vi "Load_waveform_file.vi"(10 "N":i32, 11 "Enable limit = True":bool=TRUE) -> (1 "Loop ?":i32, 2 "selected path":path, 3 "first waveform in record":waveform(dbl), 5 "Sample_Rate":dbl)   [LabVIEW 2017]
uses:
  <vilib>/Waveform/WDTFileIO.llb/Read Waveform from File.vi
  <vilib>/Waveform/WDTOps.llb/WDT Append Waveforms DBL.vi
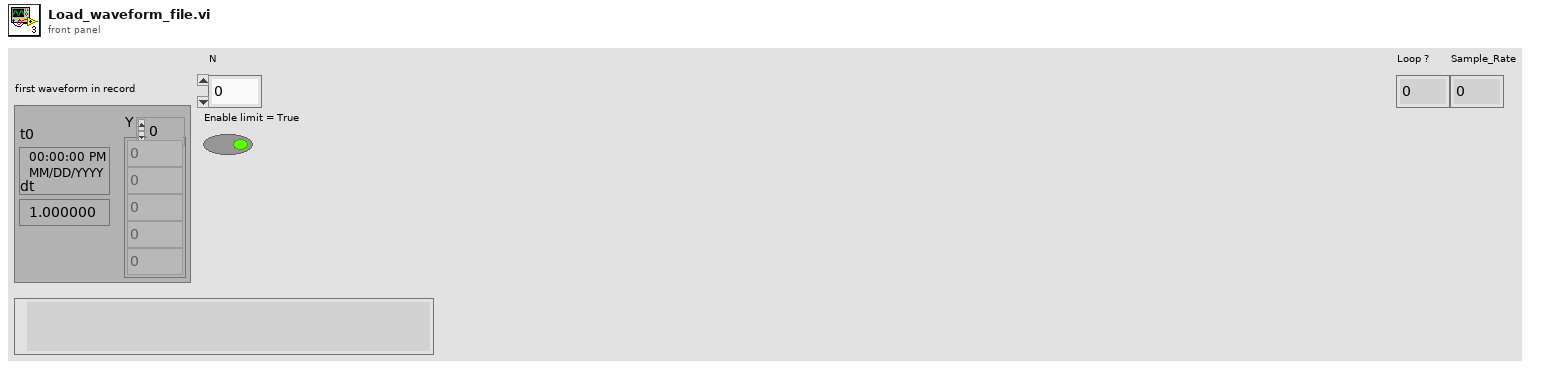
[diagram p1: front panel]
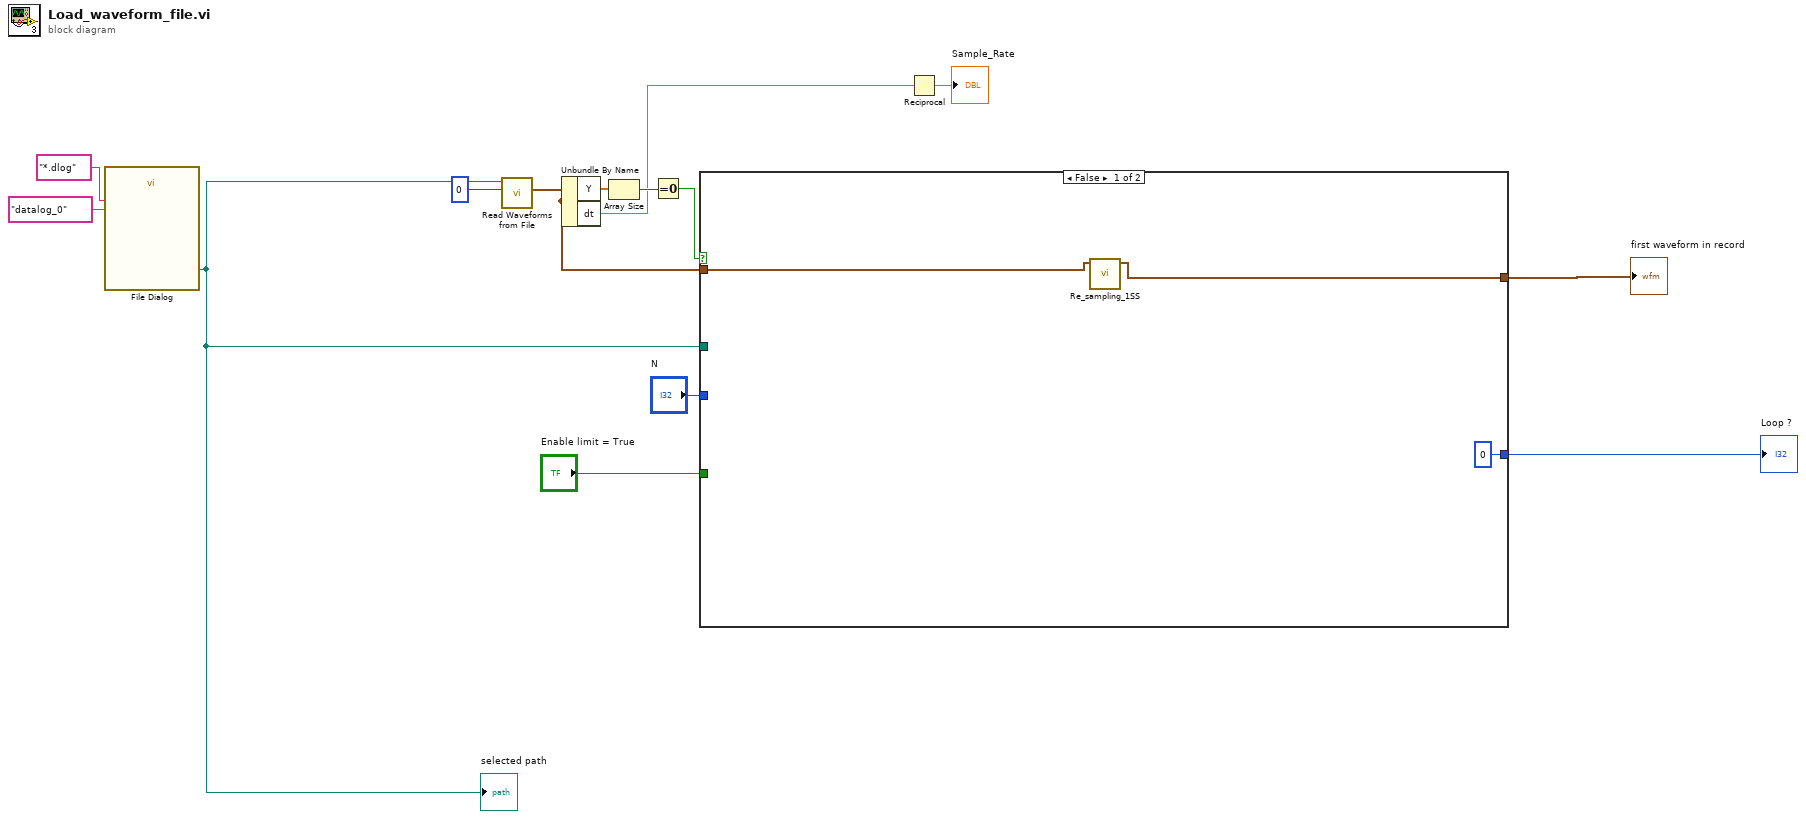
[diagram p0: block diagram]
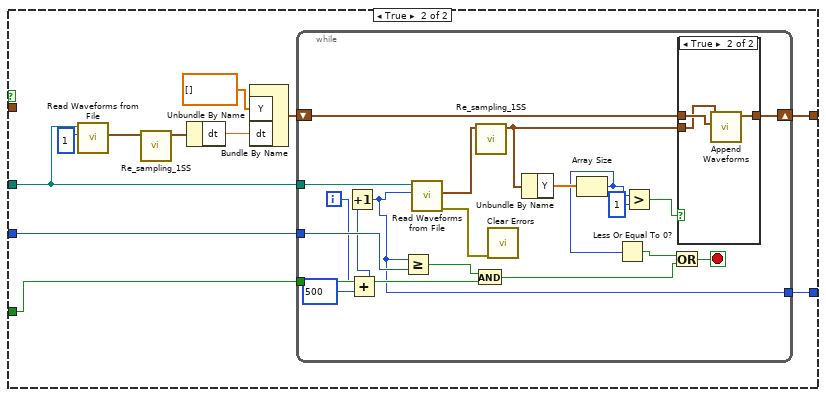
[diagram p2: hidden frame]
diagram:
  n1 = call "File Dialog"("pattern (all files)"="*.dlog", "pattern label"="datalog_0") -> ("selected path"=w11:path)  [unwired: 10 in, 3 out]
  "selected path" <- w11
  n2 = call-poly <vilib>:"Read Waveforms from File.vi"("offset (records:0)"=0, "file path (dialog if empty)"=w11) -> ("first waveform in record"=w3:waveform(dbl))  [unwired: 4 in, 3 out]
  n3 = Unbundle By Name(w3) -> ("Y"=w12:dbl[], "dt"=w2:dbl)
  n4 = Array Size(array=w12) -> (size(s)=w13:i32)
  n5 = Equal To 0?(x=w13) -> (x = 0?=w14:bool)
  n6 = case shown="False" w14 {
    tunnel: [w15 w28] -> w9
    tunnel: w11 -> [_ w23]
    tunnel: "N" -> [_ w22]
    tunnel: "Enable limit = True" -> [_ w21]
    tunnel: [0 w18] -> w4
    tunnel: w3 -> [w16 _]
    frame False {
      n7 = call "Re_sampling_1SS.vi"("Waveform_main"=w16) -> ("Waveform"=w15:waveform(dbl))  [unwired: 10 in]
    }
    frame True {
      n8 = call-poly <vilib>:"Read Waveforms from File.vi"("offset (records:0)"=1, "file path (dialog if empty)"=w23) -> ("first waveform in record"=w20:waveform(dbl))  [unwired: 4 in, 3 out]
      n9 = call "Re_sampling_1SS.vi"("Waveform_main"=w20) -> ("Waveform"=w19:waveform(dbl))  [unwired: 10 in]
      n10 = Unbundle By Name(w19) -> ("dt"=w25:dbl)
      n11 = Bundle By Name("Y"=dbl[] [], "dt"=w25) -> (w24:waveform(dbl))  [unwired: 1 in]
      n12 = while {
        shift-right: [w48] -> w28
        shift-left: w24 -> [w44]
        tunnel: w23 -> [w47]
        tunnel: w22 -> [w43]
        tunnel: w21 -> [w40]
        tunnel: [w33] -> w18
        i -> [w31]
        stop <- w42 stop-if-true
        n13 = Add(x=w31, y=500) -> (x+y=w29:i32)
        n14 = Increment(x=w29) -> (x+1=w33:i32)
        n15 = Greater Or Equal?(x=w33, y=w43) -> (x >= y?=w41:bool)
        n16 = call-poly <vilib>:"Read Waveforms from File.vi"("offset (records:0)"=w33, "file path (dialog if empty)"=w47) -> ("error out"=w45:errorcluster, "first waveform in record"=w32:waveform(dbl))  [unwired: 4 in, 2 out]
        n17 = And(x=w41, y=w40) -> (x .and. y?=w39:bool)
        n18 = call "Re_sampling_1SS.vi"("Waveform_main"=w32) -> ("Waveform"=w38:waveform(dbl))  [unwired: 10 in]
        n19 = call <vilib>:"Clear Errors.vi"("error in (no error)"=w45) -> ()  [unwired: 5 in, 2 out]
        n20 = Unbundle By Name(w38) -> ("Y"=w46:dbl[])
        n21 = Array Size(array=w46) -> (size(s)=w35:i32)
        n22 = Less Or Equal To 0?(x=w35) -> (x <= 0?=w34:bool)
        n23 = Greater?(x=w35, y=1) -> (0:w36:bool)
        n24 = Or(x=w34, y=w39) -> (x .or. y?=w42:bool)
        n25 = case shown="True" w36 {
          tunnel: [w49 w52] -> w48
          tunnel: w38 -> [_ w50]
          tunnel: w44 -> [w49 w51]
          frame False {
          }
          frame True {
            n26 = call-poly <vilib>:"Append Waveforms.vi"("waveform B"=w51, "waveform A"=w50) -> ("waveform out"=w52:waveform(dbl))  [unwired: 8 in, 1 out]
          }
        }
      }
    }
  }
  "first waveform in record" <- w9
  "Loop ?" <- w4
  n27 = Reciprocal(x=w2) -> (1/x=→"Sample_Rate":dbl)
